vi "Configure System.vi"(0 "VISA resource name":refnum<visa-resource-name>, 2 "Beeper Enabled? (T: On)":bool=TRUE, 5 "error in (no error)":errorcluster) -> (14 "VISA resource name out":refnum<visa-resource-name>, 19 "error out":errorcluster)   [LabVIEW 2020, in "Keithley 2100 Series.lvlib"]
doc: "This VI configures various system settings on the instrument. This includes enabling or disabling autozeroing and the beeper.\n\nNote:\nThis VI aborts the trigger system."
uses:
  Keithley 2100 Series.lvlib
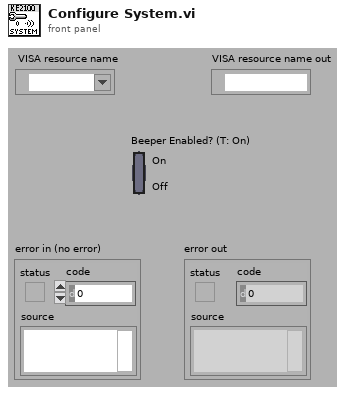
[diagram p1: front panel]
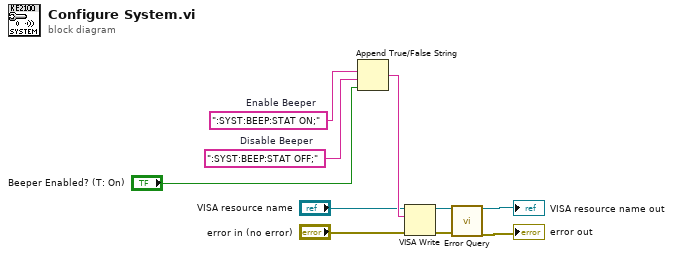
[diagram p0: block diagram]
diagram:
  w9 = ":SYST:BEEP:STAT OFF;"  # Disable Beeper
  w10 = ":SYST:BEEP:STAT ON;"  # Enable Beeper
  n1 = Append True/False String(1:"Beeper Enabled? (T: On)", 2:w9, 3:w10) -> (0:w8:string)  [unwired: 1 in]
  n2 = VISA Write(VISA resource name="VISA resource name", write buffer=w8, error in (no error)="error in (no error)") -> (VISA resource name out=w6:refnum<visa-resource-name>, error out=w5:errorcluster)  [unwired: 1 out]
  n3 = call "Error Query.vi"("VISA resource name"=w6, "error in (no error)"=w5) -> ("VISA resource name out"=→"VISA resource name out":refnum<visa-resource-name>, "error out"=→"error out":errorcluster)  [unwired: 14 in, 2 out]
